vi "JSONRPC-InvokeForJSONResult.vi"(8 "error in":errorcluster, 9 "variableArray":string[][](array[string]), 10 "variables":string, 11 "expid":string="\"%s\"") -> (0 "error out":errorcluster, 2 "responseper":string, 3 "response":string)   [LabVIEW 2020]
doc: "Parse a JSONRPC 2.0 string, invokes the corresponding method and returns only the result field of the JSON response."
panel:
  in  "method":T1(ring)=enum."get"
  # "InvokeForJSONResult"
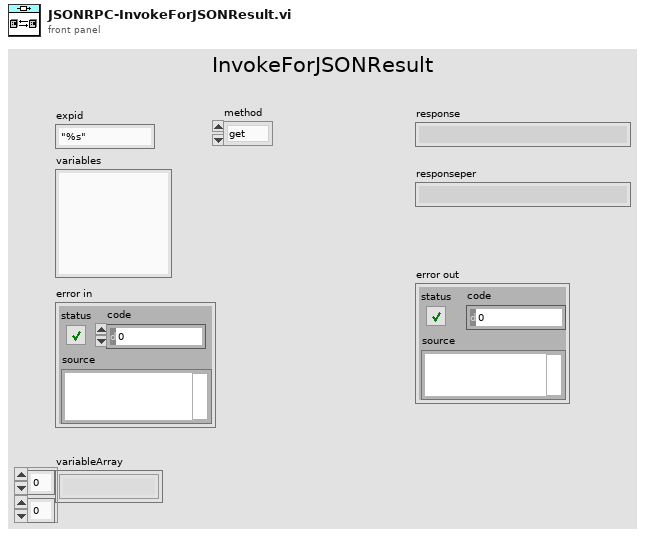
[diagram p1: front panel]
types:
  T1 = enum16{"open", "close", "start", "stop", "get", "set", "info", "UNDEFINED"}
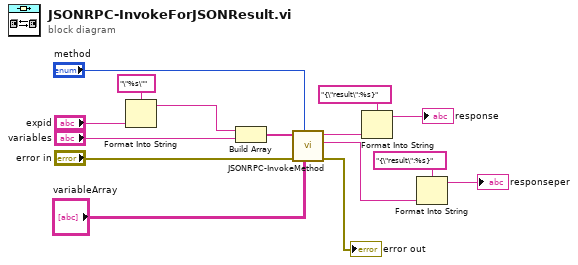
[diagram p0: block diagram]
diagram:
  n1 = Format Into String(format string="\"%s\"", "expid") -> (resulting string=w12:string)  [unwired: 2 in, 1 out]
  n2 = Build Array(w12, "variables") -> (w11:string[])
  n3 = call "JSONRPC-InvokeMethod.vi"("variableArray"="variableArray", "method"="method", "error in (no error)"="error in", "params"=w11) -> ("error out"=→"error out":errorcluster, "resultper"=w1:string, "result"=w7:string)  [unwired: 5 in]
  n4 = Format Into String(format string="{\"result\":%s}", w7) -> (resulting string=→"response":string)  [unwired: 2 in, 1 out]
  n5 = Format Into String(format string="{\"result\":%s}", w1) -> (resulting string=→"responseper":string)  [unwired: 2 in, 1 out]
